vi "Station-SeqDone.vi"(8 "error in (no error)":errorcluster, 9 "Order done (F)":bool, 10 "Status":T1, 11 "State":T2=enum."Run") -> (0 "error out":errorcluster)   [LabVIEW 2016]
uses:
  Sequence/Sequence.State.ctl
  Sequence/Sequence.Step.Status.ctl
  Station.Action.ctl
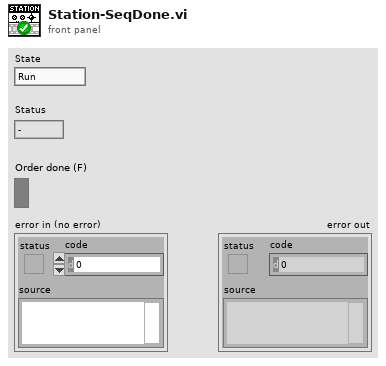
[diagram p1: front panel]
types:
  T1 = typedef "Sequence.Step.Status.ctl" = enum16{"-", "Pending", "Running", "Skipped", "Passed", "Failed", "Done", "Error", "Aborted", "Stopped"}
  T2 = typedef "Sequence.State.ctl" = enum16{"Init", "Idle", "Home", "Work", "Run", "Pause"}
  T3 = typedef "Station.Action.ctl" = enum32{"idle", "constructor", "destructor", "--- Station ---", "Hardware.Init", "Status.Update", "Status.Clear", "Order", "Init", "Ready", "Start", "Run", "Stop", "Error", "Home", "Done", "Seq.Run", "Seq.Done", "Tower.Update", "Mode.Select", "Emg", "Emg.Reset", "Emg.Check", "Home.Check", "Prod.Check", "Butt.Check"}
  T4 = cluster{"State":T2, "Status":T1, "Order done (F)":bool}
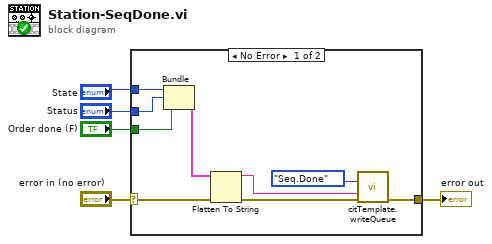
[diagram p0: block diagram]
diagram:
  n1 = case shown="No Error" "error in (no error)" {
    selector: "error in (no error)" -> [w12 w15]
    tunnel: [w14 w15] -> w5
    tunnel: "State" -> [w9 _]
    tunnel: "Status" -> [w8 _]
    tunnel: "Order done (F)" -> [w7 _]
    frame No Error {
      n2 = Bundle("State"=w9, "Status"=w8, "Order done (F)"=w7) -> (w6:T4)  [unwired: 1 in]
      n3 = Flatten To String(anything=w6, error in (no error)=w12) -> (data string=w10:string, error out=w11:errorcluster)  [unwired: 2 in, 1 out]
      n4 = call "citTemplate.writeQueue.vi"("event in (if not connected:all statemachine with data event)"=Station.Action."Seq.Done" ("Action"), "data in"=w10, "error in (no error)"=w11) -> ("error out"=w14:errorcluster)  [unwired: 12 in]
    }
    frame Error {
    }
  }
  "error out" <- w5
